vi "Split AK Name und EKFG.vi"(0 "Recipe Teil":string[][](array[string]), 11 "error in (no error)":errorcluster caption="Fehler (Eingang, kein Fehler)") -> (4 "AK Name":string[][](array[string]), 6 "AK Config Fehler":bool, 8 "EKFG":string[][](array[string]), 10 "EKFG Config Fehler":bool, 15 "error out":errorcluster caption="Fehler (Ausgang)")   [LabVIEW 2020, in "AK-Schnittstelle.lvlib"]
uses:
  AK-Schnittstelle.lvlib
  Stoerungen/Stoerungen Messgeraet/Aktionen Kommunikation Stoerung.ctl
  Stoerungen/Stoerungen.lvlib
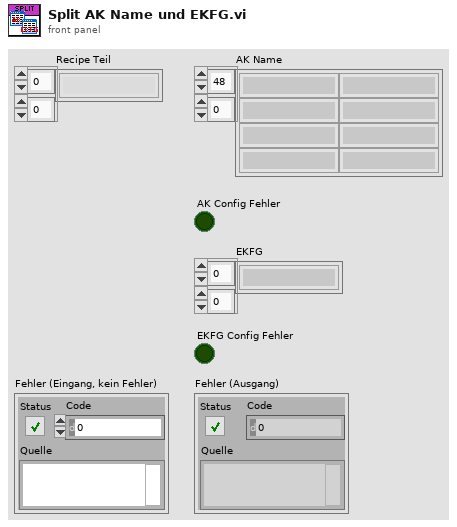
[diagram p1: front panel]
types:
  T1 = typedef "Stoerungen.lvlib/Aktionen Kommunikation Stoerung.ctl" = enum16{"lesen", "init", "FT-IR Komm", "FT-IR Betriebsart", "FT-IR Hintergrund", "cRIO Komm", "PNS Komm", "Dichtheitstest", "Life Bit", "FTIR Komm AK", "PMA Komm", "FID Komm", "PMA Cal", "FID Ch4 Cal", "FID THC Cal", "Cal Timeout", "VFS 1 Komm", "VFS 2 Komm", "VFS 3 Komm", "VFS 4 Komm", "TRE 08 Komm", "CG-Test vorzeitig", "CG-Test Span 1", "CG-Test Span 2", "CG-Test Span 3", "CG-Test Messgas", "CG-Test löschen", "Test", "Amium AK", "AK Recept konfig", "AK Name konfig", "AK EKFG konfig"}
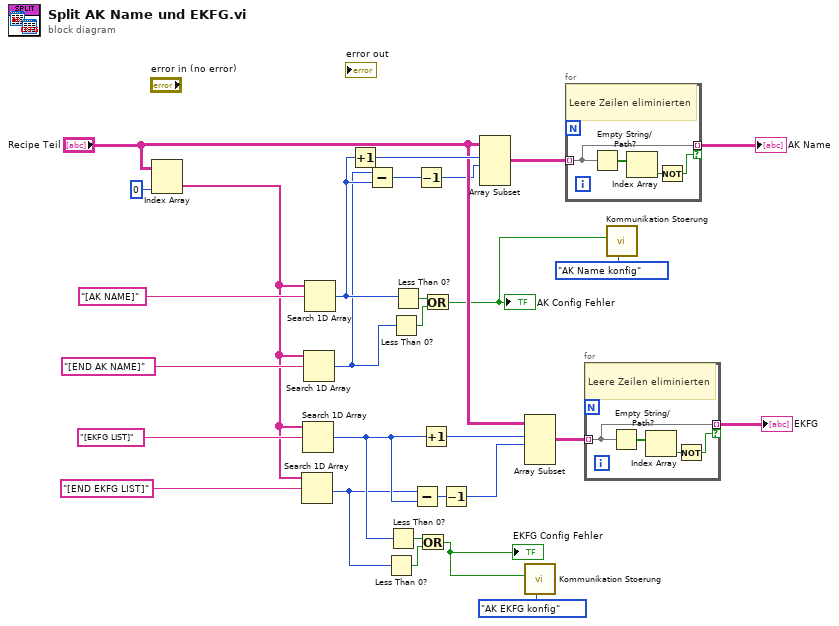
[diagram p0: block diagram]
diagram:
  n1 = Index Array(array="Recipe Teil", index (col)=0 ("Deaktivierter Index (Spalte)")) -> (element=w24:string[])  [unwired: 1 in]
  n2 = Search 1D Array(1D array=w24, element="[END EKFG LIST]" ("String")) -> (index of element=w5:i32)  [unwired: 1 in]
  n3 = Search 1D Array(1D array=w24, element="[EKFG LIST]" ("String")) -> (index of element=w6:i32)  [unwired: 1 in]
  n4 = Search 1D Array(1D array=w24, element="[END AK NAME]" ("String")) -> (index of element=w11:i32)  [unwired: 1 in]
  n5 = Search 1D Array(1D array=w24, element="[AK NAME]" ("String")) -> (index of element=w12:i32)  [unwired: 1 in]
  n6 = Increment(x=w12) -> (x+1=w22:i32)
  n7 = Subtract(x=w11, y=w12) -> (x-y=w23:i32)
  n8 = Less Than 0?(x=w5) -> (x < 0?=w8:bool)
  n9 = Less Than 0?(x=w6) -> (x < 0?=w7:bool)
  n10 = Less Than 0?(x=w11) -> (x < 0?=w9:bool)
  n11 = Less Than 0?(x=w12) -> (x < 0?=w10:bool)
  n12 = Subtract(x=w5, y=w6) -> (x-y=w20:i32)
  n13 = Decrement(x=w23) -> (x-1=w18:i32)
  n14 = Or(x=w7, y=w8) -> (x .or. y?=w1:bool)
  "EKFG Config Fehler" <- w1
  n15 = Increment(x=w6) -> (x+1=w21:i32)
  n16 = Or(x=w10, y=w9) -> (x .or. y?=w3:bool)
  "AK Config Fehler" <- w3
  n17 = Decrement(x=w20) -> (x-1=w17:i32)
  n18 = Array Subset(array="Recipe Teil", index (row)=w22, length (row)=w18) -> (w16:string[][])  [unwired: 2 in]
  n19 = Array Subset(array="Recipe Teil", index (row)=w21, length (row)=w17) -> (w14:string[][])  [unwired: 2 in]
  n20 = call "Kommunikation Stoerung.vi"("Aktionen"=Aktionen_Kommunikation_Stoerung."AK EKFG konfig", "ERROR"=w1) -> ()  [unwired: 9 in, 1 out]
  n21 = for {
    tunnel: w16 -> [w33] mode=indexing
    tunnel: [w33] -> w15 mode=indexing if=w30
    # "Leere Zeilen eliminierten"
    n22 = Empty String/Path?(string/path=w33) -> (empty?=w32:bool[])
    n23 = Index Array(array=w32) -> (element=w31:bool)  [unwired: 1 in]
    n24 = Not(x=w31) -> (.not. x?=w30:bool)
  }
  "AK Name" <- w15
  n25 = for {
    tunnel: w14 -> [w37] mode=indexing
    tunnel: [w37] -> w13 mode=indexing if=w34
    # "Leere Zeilen eliminierten"
    n26 = Empty String/Path?(string/path=w37) -> (empty?=w36:bool[])
    n27 = Index Array(array=w36) -> (element=w35:bool)  [unwired: 1 in]
    n28 = Not(x=w35) -> (.not. x?=w34:bool)
  }
  "EKFG" <- w13
  n29 = call "Kommunikation Stoerung.vi"("Aktionen"=Aktionen_Kommunikation_Stoerung."AK Name konfig", "ERROR"=w3) -> ()  [unwired: 9 in, 1 out]
